vi "ATA10003 Communicate.vi"(0 "VISA Resource In":refnum<visa-resource-name>="COM5", 1 "Function_In":string(combo)="AutoVoltage", 5 "Address(0x01)":u8=1 format="%.0x", 7 "Value":dbl=264.0, 11 "error in (no error)":errorcluster) -> (4 "VISA Resource Out":refnum<visa-resource-name>, 6 "OK ?":bool, 8 "Value":dbl, 10 "Return String":string, 15 "error out":errorcluster)   [LabVIEW 2015]
uses:
  Instance           2 37Saved   AC PS Set Voltage & Frequency .vi
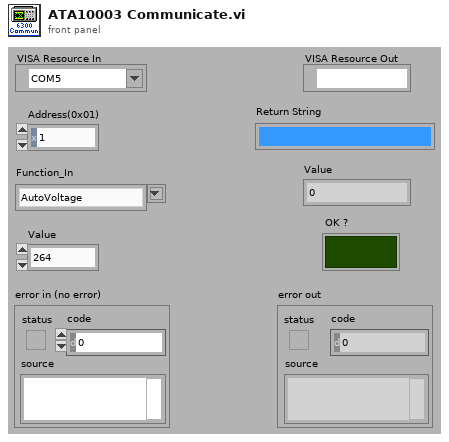
[diagram p1: front panel]
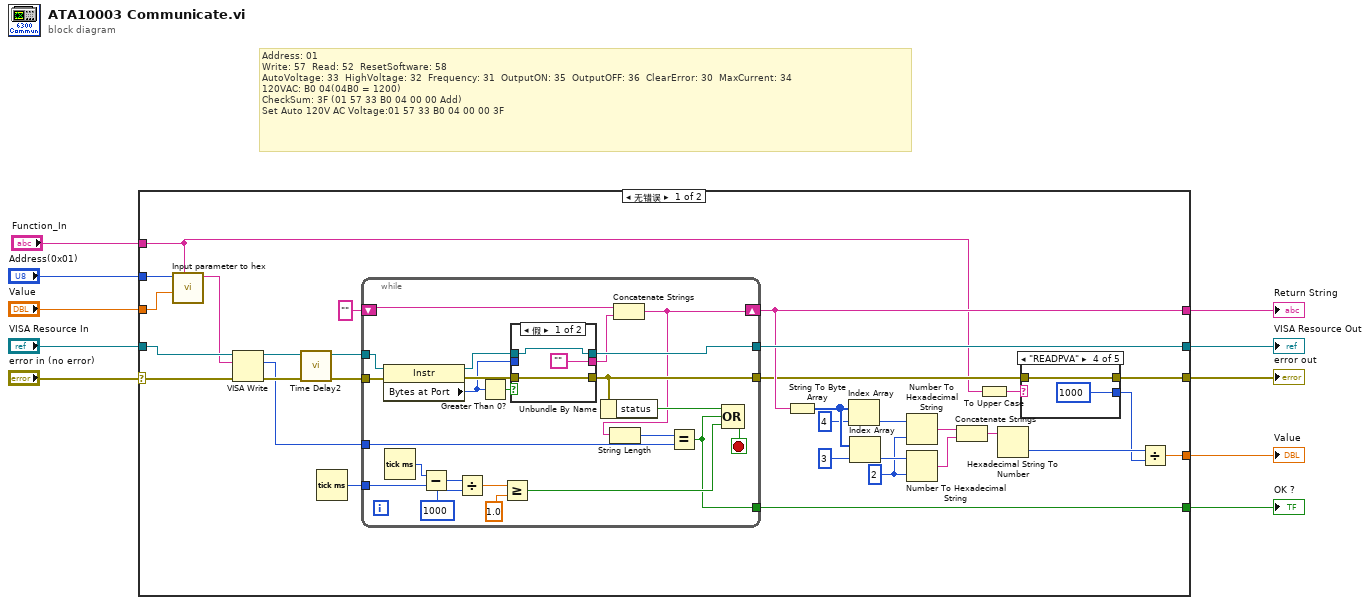
[diagram p0: block diagram]
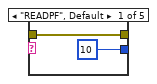
[diagram p2: hidden frame]
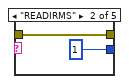
[diagram p3: hidden frame]
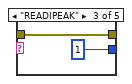
[diagram p4: hidden frame]
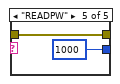
[diagram p5: hidden frame]
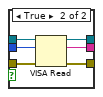
[diagram p6: hidden frame]
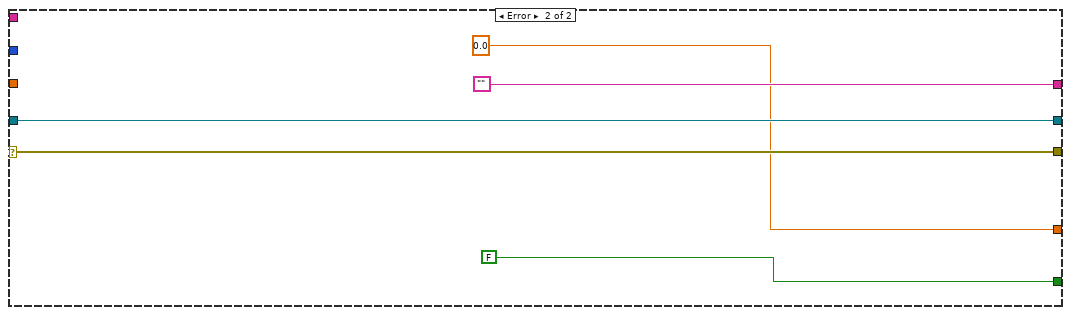
[diagram p7: hidden frame]
diagram:
  # "Address: 01\nWrite: 57  Read: 52  ResetSoftware: 58\nAutoVoltage: 33  HighVoltage: 32  Frequency: 31  OutputON: 35  OutputOFF: 36  ClearError: 30  MaxCurrent: 34\n120VAC: B0 04(04B0 = 1200)\nCheckSum: 3F (01 57 33 B0 04 00 00 Add)\nSet Auto 120V AC Voltage:01 57 33 B0 04 00 00 3F"
  n1 = case shown="无错误" "error in (no error)" {
    selector: "error in (no error)" -> [w40 w87]
    tunnel: [w15 w87] -> w5
    tunnel: [w38 w86] -> w6
    tunnel: "VISA Resource In" -> [w39 w86]
    tunnel: [w17 FALSE] -> w8
    tunnel: [w19 ""] -> w7
    tunnel: "Address(0x01)" -> [w32 _]
    tunnel: "Value" -> [w31 _]
    tunnel: "Function_In" -> [w14 _]
    tunnel: [w18 0.0] -> w1
    frame No Error {
      w11 = i16 2 ("width (-)")
      n2 = call "Input parameter to hex.vi"("Function_In"=w14, "Value"=w31, "Address(0x01)"=w32) -> ("Command(hex)"=w30:string)  [unwired: 8 in]
      n3 = VISA Write(VISA resource name=w39, write buffer=w30, error in (no error)=w40) -> (VISA resource name out=w33:refnum<visa-resource-name>, return count=w29:u32, error out=w34:errorcluster)
      n4 = call "Time Delay2"("error in (no error)"=w34) -> ("error out"=w36:errorcluster)  [unwired: 10 in]
      n5 = Tick Count (ms)() -> (millisecond timer value=w37:u32)
      n6 = while {
        tunnel: w33 -> [w73]
        tunnel: [w68] -> w38
        tunnel: [w67] -> w16
        tunnel: w37 -> [w60]
        tunnel: [w55] -> w17
        tunnel: w36 -> [w57]
        shift-right: [w54] -> w19
        shift-left: "" -> [w52]
        tunnel: w29 -> [w51]
        stop <- w65 stop-if-true
        n7 = property class="Instr"(reference=w73, error in=w57) -> (reference out=w71:refnum<visa-resource-name>, error out=w72:errorcluster, "Bytes at Port"=w70:u32)
        n8 = Tick Count (ms)() -> (millisecond timer value=w64:u32)
        n9 = Subtract(x=w64, y=w60) -> (x-y=w61:u32)
        n10 = Divide(x=w61, y=u32 1000) -> (x/y=w63:dbl)
        n11 = Greater Than 0?(x=w70) -> (x > 0?=w69:bool)
        n12 = Greater Or Equal?(x=w63, y=1.0) -> (x >= y?=w58:bool)
        n13 = case shown="假" w69 {
          tunnel: w72 -> [w74 w82]
          tunnel: w71 -> [w75 w81]
          tunnel: w70 -> [_ w80]
          tunnel: [w74 w79] -> w67
          tunnel: [w75 w78] -> w68
          tunnel: ["" w77] -> w53
          frame False {
          }
          frame True {
            n14 = VISA Read(VISA resource name=w81, byte count=w80, error in (no error)=w82) -> (VISA resource name out=w78:refnum<visa-resource-name>, read buffer=w77:string, error out=w79:errorcluster)  [unwired: 1 out]
          }
        }
        n15 = Unbundle By Name(w67) -> ("status"=w66:bool)
        n16 = Concatenate Strings(w52, w53) -> (w54:string)
        n17 = String Length(string=w54) -> (length=w56:i32)
        n18 = Equal?(x=w56, y=w51) -> (x = y?=w55:bool)
        n19 = Compound Arithmetic op=OR(w66, w55, w58) -> (w65:bool)
      }
      n20 = String To Byte Array(string=w19) -> (unsigned byte array=w28:u8[])
      n21 = Index Array(array=w28, index=4) -> (element=w22:u8)
      n22 = Index Array(array=w28, index=3) -> (element=w23:u8)
      n23 = Number To Hexadecimal String(1:w11, 2:w22) -> (0:w24:string)
      n24 = Number To Hexadecimal String(1:w11, 2:w23) -> (0:w25:string)
      n25 = Concatenate Strings(w24, w25) -> (w26:string)
      n26 = To Upper Case(1:w14) -> (0:w12:string)
      n27 = Hexadecimal String To Number(string=w26) -> (number=w27:u32)  [unwired: 2 in, 1 out]
      n28 = case shown="\"READPVA\"" w12 {
        tunnel: w16 -> [w42 w44 w46 w48 w50]
        tunnel: [w42 w44 w46 w48 w50] -> w15
        tunnel: [u32 10 ("y") u32 1 ("y") u32 1 ("y") u32 1000 ("y") u32 1000 ("y")] -> w13
        frame "READPF", Default {
        }
        frame "READIRMS" {
        }
        frame "READIPEAK" {
        }
        frame "READPVA" {
        }
        frame "READPW" {
        }
      }
      n29 = Divide(x=w27, y=w13) -> (x/y=w18:dbl)
    }
    frame Error {
    }
  }
  "error out" <- w5
  "VISA Resource Out" <- w6
  "OK ?" <- w8
  "Return String" <- w7
  "Value" <- w1
